vi "Start Tracking.vi"(8 "error in (no error)":errorcluster, 10 "Tracker Type":refnum<class "Data Tracker Msg.lvclass">, 11 "Data Tracker in":refnum<class "Data Tracker.lvclass">) -> (0 "error out":errorcluster, 3 "Data Tracker out":refnum<class "Data Tracker.lvclass">)   [LabVIEW 2020, in "Data Tracker.lvlib" / "Data Tracker.lvclass"]
doc: "Add a Tracker Element to the Data Tracker and setup a subscription for the Data types if needed."
uses:
  Data Tracker.lvclass
  Messages for this Actor/Data Tracker Msg/Data Tracker Msg.lvclass
  Data Tracker.lvclass/Data Tracker.ctl
  Controls/Ctl_Tracker Element.ctl
  PPL/HDH.Data.Generic.lvlibp/Data.lvclass
  PPL/HDH.Actor Framework.Core.Actor.lvlibp/1abvi3w/vi.lib/ActorFramework/Message Enqueuer/Message Priority.ctl
  PPL/HDH.Actor Framework.Core.Publisher.lvlibp/Publisher Messages/Subscribe Msg/Subscribe Msg.lvclass
  PPL/HDH.Actor Framework.Core.Actor.lvlibp/1abvi3w/vi.lib/ActorFramework/Message Enqueuer/Message Enqueuer.lvclass
  C:/Current projects/WS/PPL/HDH.Actor Framework.Core.Actor.lvlibp/1abvi3w/vi.lib/ActorFramework/Actor/Actor.lvclass
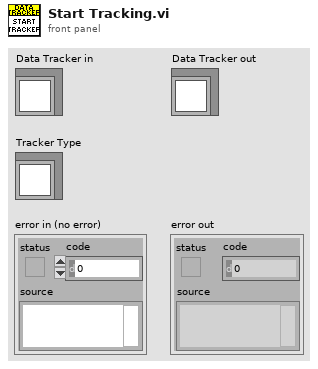
[diagram p1: front panel]
types:
  T1 = typedef "HDH.Actor Framework.Core.Actor.lvlibp/Message Enqueuer.lvclass/Message Priority.ctl" = enum16{"Low", "Normal", "High"}
  T2 = typedef "Data Tracker.lvlib/Data Tracker.lvclass/Ctl_Tracker Element.ctl" = cluster{"Tracker Type":refnum<class "Data Tracker Msg.lvclass">, "Subscriptions":refnum<class "Data.lvclass">[], "Data":refnum<class "Data.lvclass">[], "Size":u32, "Start Time":timestamp}
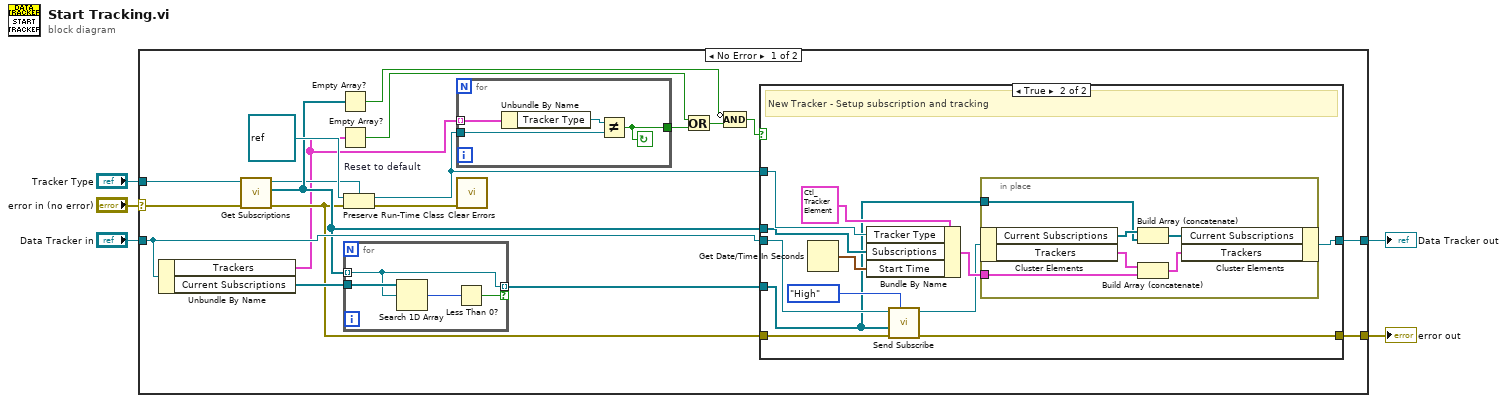
[diagram p0: block diagram]
diagram:
  n1 = case shown="No Error" "error in (no error)" {
    selector: "error in (no error)" -> [w11 w54]
    tunnel: [w18 w54] -> w4
    tunnel: [w20 w53] -> w2
    tunnel: "Data Tracker in" -> [w21 w53]
    tunnel: "Tracker Type" -> [w13 _]
    frame No Error {
      n2 = Unbundle By Name(w21) -> ("Trackers"=w9:T2[], "Current Subscriptions"=w22:refnum<class "Data.lvclass">[])
      n3 = call-dynamic "Get Subscriptions.vi"("error in (no error)"=w11, "Data Tracker Msg in"=w13) -> ("error out"=w10:errorcluster, "Subscriptions"=w15:refnum<class "Data.lvclass">[], "Data Tracker Msg out"=w12:refnum<class "Data Tracker Msg.lvclass">)  [unwired: 7 in]
      n4 = Empty Array?(array=w15) -> (empty?=w17:bool)
      n5 = Empty Array?(array=w9) -> (empty?=w8:bool)
      n6 = Preserve Run-Time Class "Reset to default"(object in=refnum<class> refnum ("LabVIEW Object"), error in=w10, 2:w12) -> (object out=w14:refnum<class "Data Tracker Msg.lvclass">, error out=w23:errorcluster)
      n7 = for {
        tunnel: w15 -> [w26] mode=indexing
        tunnel: w22 -> [w28]
        tunnel: [w26] -> w19 mode=indexing if=w25
        n8 = Search 1D Array(1D array=w28, element=w26) -> (index of element=w27:i32)  [unwired: 1 in]
        n9 = Less Than 0?(x=w27) -> (x < 0?=w25:bool)
      }
      n10 = for {
        tunnel: w9 -> [w52] mode=indexing
        tunnel: w14 -> [w50]
        tunnel: [w49] -> w7
        stop <- w49 continue-if-true
        n11 = Unbundle By Name(w52) -> ("Tracker Type"=w51:refnum<class "Data Tracker Msg.lvclass">)
        n12 = Not Equal?(x=w51, y=w50) -> (x != y?=w49:bool)
      }
      n13 = call <vilib>:"Clear Errors.vi"("error in (no error)"=w23) -> ()  [unwired: 5 in, 2 out]
      n14 = Or(x=w8, y=w7) -> (x .or. y?=w6:bool)
      n15 = Compound Arithmetic op=AND(invert w17, w6) -> (w16:bool)
      n16 = case shown="True" w16 {
        tunnel: [w30 w38] -> w20
        tunnel: w21 -> [w30 w37]
        tunnel: w14 -> [_ w41]
        tunnel: w15 -> [_ w32]
        tunnel: w19 -> [_ w31]
        tunnel: [w29 w33] -> w18
        tunnel: w10 -> [w29 w34]
        frame False {
          # "Already tracking - Abort"
        }
        frame True {
          # "New Tracker - Setup subscription and tracking"
          n17 = Get Date/Time In Seconds() -> (seconds since 1Jan1904=w40:timestamp)
          n18 = Bundle By Name(cluster=T2 {"Tracker Type"=refnum, "Subscriptions"=[], "Data"=[], "Size"=0, "Start Time"=timestamp(0 s since 1904-01-01)} ("Tracker Element"), "Tracker Type"=w41, "Subscriptions"=w32, "Start Time"=w40) -> (w39:T2)
          n19 = call "Send Subscribe.vi"("Message Priority (High)"=Message_Priority."High", "error in (no error)"=w34, "Data Array"=w31, "Actor in"=w37) -> ("error out"=w33:errorcluster, "Actor out"=w36:refnum<class "Data Tracker.lvclass">)  [unwired: 6 in]
          n20 = in-place {
            in-place-border: w31 -> [w47]
            in-place-border: w39 -> [w44]
            n21 = in-place-cluster #1(w36) -> ("Current Subscriptions"=w48:refnum<class "Data.lvclass">[], "Trackers"=w45:T2[])
            n22 = Build Array (concatenate)(w48, w47) -> (w46:refnum<class "Data.lvclass">[])
            n23 = Build Array (concatenate)(w45, w44) -> (w43:T2[])
            n24 = in-place-cluster #1("Current Subscriptions"=w46, "Trackers"=w43) -> (w38:refnum<class "Data Tracker.lvclass">)
          }
        }
      }
    }
    frame Error {
    }
  }
  "error out" <- w4
  "Data Tracker out" <- w2
